vi "Read Forward RF Power.vi"(8 "error in (no error)":errorcluster, 11 "Comdel in":refnum<class "PL Comdel CX.lvclass">) -> (0 "error out":errorcluster, 2 "power, W":u16, 3 "Comdel out":refnum<class "PL Comdel CX.lvclass">)   [LabVIEW 2015, in "PL Comdel CX.lvclass"]
doc: "Reads forward RF power."
uses:
  PL Comdel CX.lvclass
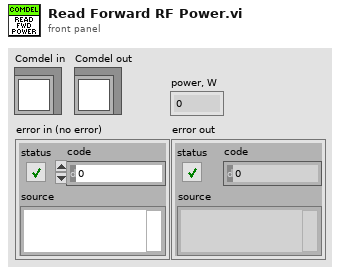
[diagram p1: front panel]
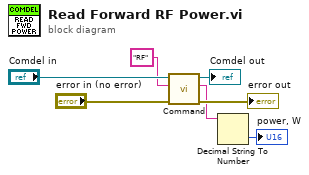
[diagram p0: block diagram]
diagram:
  n1 = call "Command.vi"("error in (no error)"="error in (no error)", "command"="RF", "Comdel in"="Comdel in") -> ("error out"=→"error out":errorcluster, "response data"=w2:string, "Comdel out"=→"Comdel out":refnum<class "PL Comdel CX.lvclass">)  [unwired: 6 in]
  n2 = Decimal String To Number(string=w2) -> (number=→"power, W":i32)  [unwired: 2 in, 1 out]
